vi "test_generic.vi"() -> ()   [LabVIEW 2010, in "GenericSignalReader.lvclass"]
uses:
  GenericSignalReader.lvclass
  Clock/GenericClock/GenericClock/GenericClock.lvclass
  common/classes/GenericComponent/GenericComponent/GenericComponent.lvclass
  main/labview_source/type_definitions/enumerations/run_mode_enum.ctl
panel:
  in  "continuous?":bool
  out "signals":dbl[][](graph)
  out "buffer overflow?":bool
  in  "block size":i32=10000
  out "event loop counter":i32
  in  "sample clock frequency":dbl[unit]=40000.0
  in  "number of samples":i32=1000000000
  in  "Clock createButton":bool caption="createButton"
  in  "SignalReader createButton":bool caption="createButton"
  in  "startReadingButton":bool
  in  "stopButton":bool
  # "Test Suite for SignalReader components"
  # "How to use this Test Suite\n\n1. Choose your SignalReader component path.\n2. Select the configuration for your SignalReader.\n3. Create the SignalReader instance.\n4. Choose the Clock component path.\n5. Select the configuration for the Clock.\n6. Start the reading process."
  # "SignalReader"
  # "Clock"
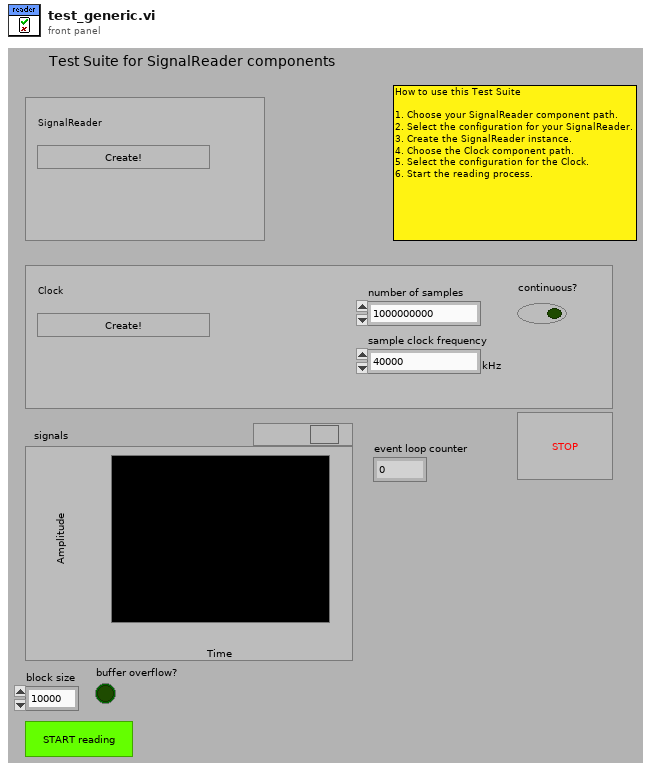
[diagram p1: front panel]
types:
  T1 = typedef "run_mode_enum.ctl" = enum16{"focus mode", "single sweep mode", "experiment mode"}
  T2 = typedef "XComponentSpecification.xctl/data.ctl" = cluster{"class path":string, "configuration":string, "label":string, "settings name":string}
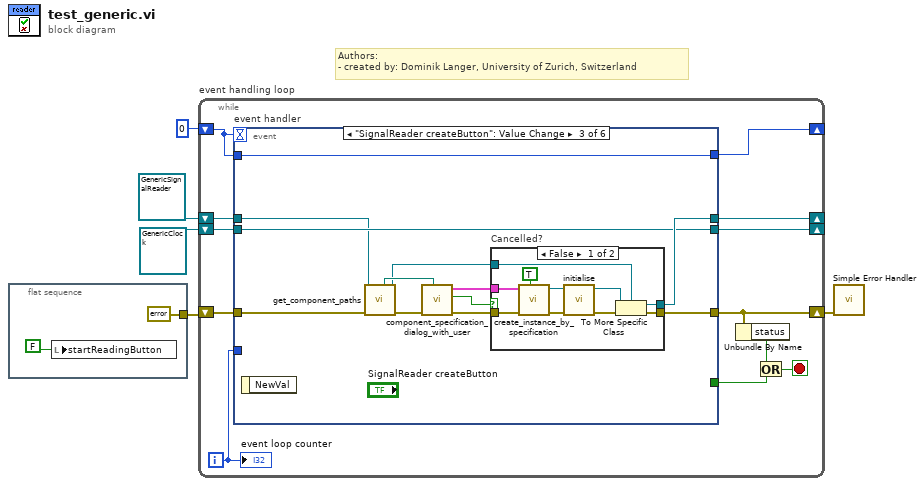
[diagram p0: block diagram]
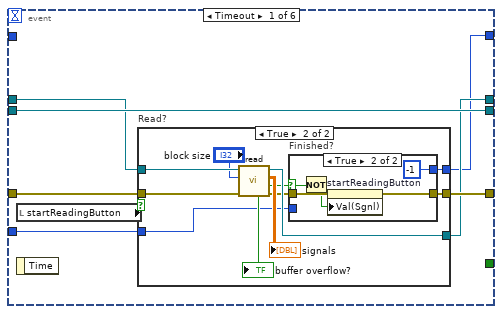
[diagram p2: hidden frame]
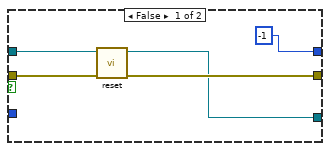
[diagram p3: hidden frame]
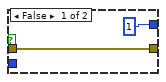
[diagram p4: hidden frame]
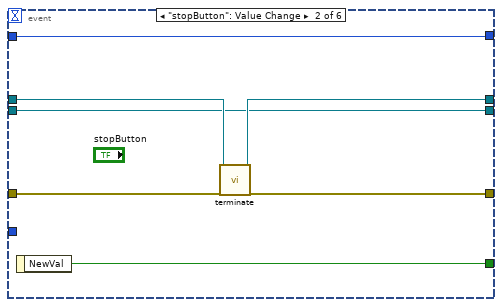
[diagram p5: hidden frame]
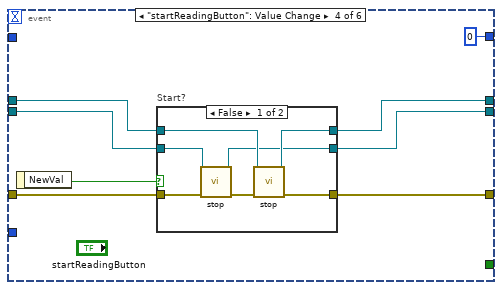
[diagram p7: hidden frame]
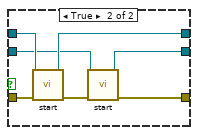
[diagram p8: hidden frame]
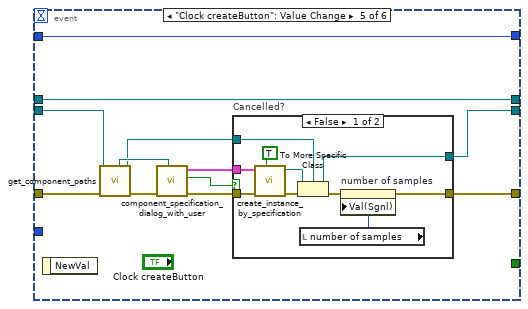
[diagram p9: hidden frame]
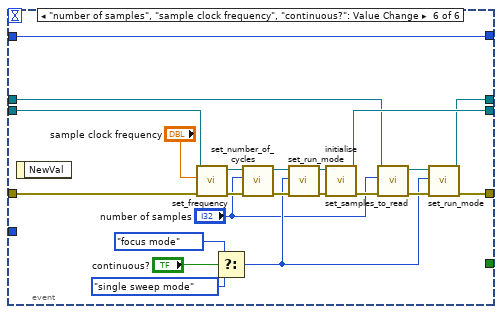
[diagram p11: hidden frame]
diagram:
  # "Authors: \n- created by: Dominik Langer, University of Zurich, Switzerland"
  n1 = flat-sequence {
    tunnel: [errorcluster {"status"=FALSE, "code"=0, "source"=""} ("error out")] -> w3
    frame #0 {
      n2 = local write "startReadingButton"(FALSE ("startClockButton")) -> ()
    }
  }
  n3 = while "event handling loop" {
    shift-right: [w16] -> w5
    shift-left: w3 -> [w19]
    shift-right: [w17] -> _
    shift-left: refnum<class "GenericSignalReader.lvclass"> refnum ("GenericSignalReader.lvclass") -> [w18]
    shift-right: [w11] -> _
    shift-left: refnum<class "GenericClock.lvclass"> refnum ("GenericClock.lvclass") -> [w12]
    shift-right: [w9] -> _
    shift-left: 0 -> [w10]
    i -> [w8]
    stop <- w13 stop-if-true
    n4 = event "event handler" shown="[2] \"SignalReader createButton\": Value Change" {
      selector: _ -> [_ _ _ _ _ _]
      dyn-events: _ -> [_ _ _ _ _ _]
      timeout: w10 -> [_ _ _ _ _ _]
      tunnel: w19 -> [w26 w57 w63 w89 w110 w149]
      tunnel: [w25 w56 w69 w88 w113 w139] -> w16
      tunnel: w18 -> [w24 w55 w61 w87 w115 w141]
      tunnel: [w23 w54 w68 w86 w115 w137] -> w17
      tunnel: [_ w53 _ _ _ _] -> w14
      tunnel: w12 -> [w27 w52 w67 w84 w108 w145]
      tunnel: [w27 w52 w67 w83 w106 w144] -> w11
      tunnel: [w22 w51 w66 0 w114 w143] -> w9
      tunnel: w10 -> [_ w51 w66 _ w114 w143]
      tunnel: w8 -> [w20 _ _ _ _ _]
      event Timeout {
        n5 = local read "startReadingButton"() -> (w21:bool)
        n6 = event-data() -> ()  [unwired: 1 in, 1 out]
        n7 = case "Read?" shown="True" w21 {
          tunnel: w26 -> [w31 w43]
          tunnel: [w28 w42] -> w23
          tunnel: w24 -> [w29 w40]
          tunnel: [w30 w35] -> w25
          tunnel: [-1 w37] -> w22
          tunnel: w20 -> [_ w33]
          frame False {
            n8 = call-dynamic "reset.vi"("error in (no error)"=w31, "GenericSignalReader in"=w29) -> ("error out"=w30:errorcluster, "GenericSignalReader out"=w28:refnum<class "GenericSignalReader.lvclass">)  [unwired: 8 in]
          }
          frame True {
            n9 = call-dynamic "read.vi"("error in (no error)"=w43, "block size"="block size", "SignalReader in"=w40) -> ("error out"=w36:errorcluster, "finished?"=w34:bool, "signals read"=→"signals":dbl[][], "SignalReader out"=w42:refnum<class "GenericSignalReader.lvclass">, "buffer overflow?"=→"buffer overflow?":bool)  [unwired: 4 in]
            n10 = case "Finished?" shown="True" w34 {
              selector: w34 -> [_ w47]
              tunnel: [1 -1] -> w37
              tunnel: w36 -> [w45 w49]
              tunnel: [w45 w48] -> w35
              tunnel: w33 -> [_ _]
              frame False {
              }
              frame True {
                n11 = Not(x=w47) -> (.not. x?=w46:bool)
                n12 = property on="startReadingButton" class="Bool (strict)"(error in=w49, "Val(Sgnl)"=w46) -> (error out=w48:errorcluster)  [unwired: 1 in, 1 out]
              }
            }
          }
        }
      }
      event "stopButton": Value Change {
        n13 = event-data() -> ("NewVal"=w53:bool)  [unwired: 1 in]
        n14 = call-dynamic "terminate.vi"("error in (no error)"=w57, "GenericPlugin in"=w55) -> ("error out"=w56:errorcluster, "GenericPlugin out"=w54:refnum<class "GenericSignalReader.lvclass">)  [unwired: 8 in]
      }
      event "SignalReader createButton": Value Change {
        n15 = event-data() -> ()  [unwired: 1 in, 1 out]
        n16 = call-dynamic "get_component_paths.vi"("error in (no error)"=w63, "GenericComponent in"=w61) -> ("error out"=w64:errorcluster, "GenericComponent out"=w60:refnum<class "GenericSignalReader.lvclass">, "component type directory"=w65:path)  [unwired: 4 in, 3 out]
        n17 = call "component_specification_dialog_with_user.vi"("start path"=w65, "error in (no error)"=w64) -> ("error out"=w62:errorcluster, "cancelled?"=w59:bool, "component specification out"=w58:T2)  [unwired: 7 in]
        n18 = case "Cancelled?" shown="False" w59 {
          tunnel: [w79 w81] -> w69
          tunnel: [w78 w80] -> w68
          tunnel: w62 -> [w72 w81]
          tunnel: w60 -> [w71 w80]
          tunnel: w58 -> [w70 _]
          frame False {
            n19 = call "create_instance_by_specification.vi"("call constructor?"=TRUE, "error in (no error)"=w72, "component specification"=w70) -> ("error out"=w75:errorcluster, "GenericPlugin out"=w74:refnum<class "GenericComponent.lvclass">)  [unwired: 6 in, 1 out]
            n20 = call-dynamic "initialise.vi"("error in (no error)"=w75, "GenericPlugin in"=w74) -> ("error out"=w76:errorcluster, "GenericPlugin out"=w77:refnum<class "GenericComponent.lvclass">)  [unwired: 8 in]
            n21 = To More Specific Class(target class=w71, reference=w77, error in=w76) -> (specific class reference=w78:refnum<class "GenericSignalReader.lvclass">, error out=w79:errorcluster)
          }
          frame True {
          }
        }
      }
      event "startReadingButton": Value Change {
        n22 = event-data() -> ("NewVal"=w85:bool)  [unwired: 1 in]
        n23 = case "Start?" shown="False" w85 {
          tunnel: w89 -> [w93 w103]
          tunnel: [w94 w99] -> w88
          tunnel: w87 -> [w96 w102]
          tunnel: [w95 w101] -> w86
          tunnel: w84 -> [w91 w98]
          tunnel: [w90 w97] -> w83
          frame False {
            n24 = call-dynamic "stop.vi"("error in (no error)"=w93, "GenericClock in"=w91) -> ("error out"=w92:errorcluster, "GenericClock out"=w90:refnum<class "GenericClock.lvclass">)  [unwired: 8 in]
            n25 = call-dynamic "stop.vi"("error in (no error)"=w92, "GenericSignalReader in"=w96) -> ("error out"=w94:errorcluster, "GenericSignalReader out"=w95:refnum<class "GenericSignalReader.lvclass">)  [unwired: 8 in]
          }
          frame True {
            n26 = call-dynamic "start.vi"("error in (no error)"=w103, "GenericSignalReader in"=w102) -> ("error out"=w100:errorcluster, "GenericSignalReader out"=w101:refnum<class "GenericSignalReader.lvclass">)  [unwired: 8 in]
            n27 = call-dynamic "start.vi"("error in (no error)"=w100, "GenericClock in"=w98) -> ("error out"=w99:errorcluster, "GenericClock out"=w97:refnum<class "GenericClock.lvclass">)  [unwired: 8 in]
          }
        }
      }
      event "Clock createButton": Value Change {
        n28 = event-data() -> ()  [unwired: 1 in, 1 out]
        n29 = call-dynamic "get_component_paths.vi"("error in (no error)"=w110, "GenericComponent in"=w108) -> ("error out"=w111:errorcluster, "GenericComponent out"=w107:refnum<class "GenericClock.lvclass">, "component type directory"=w112:path)  [unwired: 4 in, 3 out]
        n30 = call "component_specification_dialog_with_user.vi"("start path"=w112, "error in (no error)"=w111) -> ("error out"=w109:errorcluster, "cancelled?"=w105:bool, "component specification out"=w104:T2)  [unwired: 7 in]
        n31 = case "Cancelled?" shown="False" w105 {
          tunnel: [w124 w126] -> w113
          tunnel: w109 -> [w119 w126]
          tunnel: w107 -> [w118 w127]
          tunnel: [w117 w127] -> w106
          tunnel: w104 -> [w116 _]
          frame False {
            n32 = call "create_instance_by_specification.vi"("call constructor?"=TRUE, "error in (no error)"=w119, "component specification"=w116) -> ("error out"=w121:errorcluster, "GenericPlugin out"=w120:refnum<class "GenericComponent.lvclass">)  [unwired: 6 in, 1 out]
            n33 = To More Specific Class(target class=w118, reference=w120, error in=w121) -> (specific class reference=w117:refnum<class "GenericClock.lvclass">, error out=w125:errorcluster)
            n34 = local read "number of samples"() -> (w123:i32)
            n35 = property on="number of samples" class="DigNum (strict)"(error in=w125, "Val(Sgnl)"=w123) -> (error out=w124:errorcluster)  [unwired: 1 in, 1 out]
          }
          frame True {
          }
        }
      }
      event "number of samples", "sample clock frequency", "continuous?": Value Change {
        n36 = event-data() -> ()  [unwired: 1 in, 1 out]
        n37 = call-dynamic "set_frequency.vi"("error in (no error)"=w149, "frequency"="sample clock frequency", "GenericClock.lvclass in"=w145) -> ("error out"=w147:errorcluster, "GenericClock.lvclass out"=w146:refnum<class "GenericClock.lvclass">)  [unwired: 7 in]
        n38 = Select(t=run_mode_enum."focus mode", s="continuous?", f=run_mode_enum."single sweep mode" ("run mode")) -> (s? t:f=w129:T1)
        n39 = call-dynamic "set_number_of_cycles.vi"("error in (no error)"=w147, "number of cycles"="number of samples", "GenericClock.lvclass in"=w146) -> ("error out"=w133:errorcluster, "GenericClock.lvclass out"=w132:refnum<class "GenericClock.lvclass">)  [unwired: 7 in]
        n40 = call-dynamic "set_run_mode.vi"("error in (no error)"=w133, "run mode"=w129, "GenericPlugin in"=w132) -> ("error out"=w130:errorcluster, "GenericPlugin out"=w131:refnum<class "GenericClock.lvclass">)  [unwired: 7 in]
        n41 = call-dynamic "initialise.vi"("error in (no error)"=w130, "GenericPlugin in"=w131) -> ("error out"=w142:errorcluster, "GenericPlugin out"=w144:refnum<class "GenericClock.lvclass">)  [unwired: 8 in]
        n42 = call-dynamic "set_samples_to_read.vi"("error in (no error)"=w142, "samples to read"="number of samples", "GenericSignalReader in"=w141) -> ("error out"=w140:errorcluster, "GenericSignalReader out"=w138:refnum<class "GenericSignalReader.lvclass">)  [unwired: 7 in]
        n43 = call-dynamic "set_run_mode.vi"("error in (no error)"=w140, "run mode"=w129, "GenericPlugin in"=w138) -> ("error out"=w139:errorcluster, "GenericPlugin out"=w137:refnum<class "GenericSignalReader.lvclass">)  [unwired: 7 in]
      }
    }
    n44 = Unbundle By Name(w16) -> ("status"=w15:bool)
    n45 = Or(x=w15, y=w14) -> (x .or. y?=w13:bool)
    "event loop counter" <- w8
  }
  n46 = call <vilib>:"Simple Error Handler.vi"("error in (no error)"=w5) -> ()  [unwired: 4 in, 5 out]
